vi "Execute Or Recurse.vi"(7 "Actor in":refnum<class "Actor.lvclass">, 8 "Error in":errorcluster, 10 "Msg":refnum<class "Msg.lvclass">) -> (0 "Error out":errorcluster, 2 "Msg Output":refnum<class "Msg Output.lvclass">, 5 "Actor out":refnum<class "Actor.lvclass">)   [LabVIEW 2025, in "jettl.lvlib"]
uses:
  jettl.lvlib
  Msg/Msg.lvclass
  Actor/Actor.lvclass
  Msg Output/Msg Output.lvclass
  Default Implementation.vi
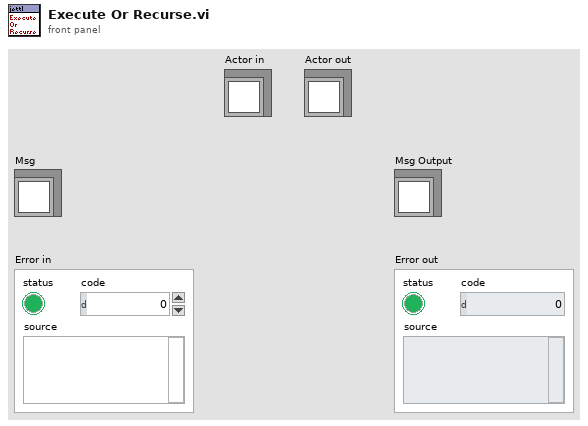
[diagram p1: front panel]
types:
  T1 = typedef "jettl.lvlib/Msgs.ctl" = set{refnum<class "Msg.lvclass">}
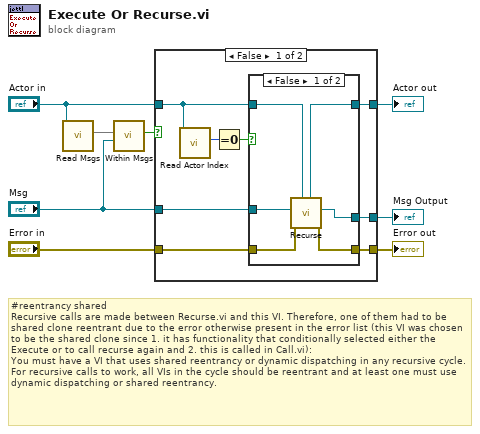
[diagram p0: block diagram]
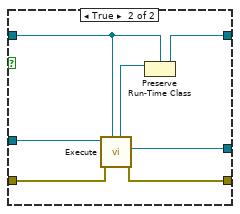
[diagram p3: hidden frame]
diagram:
  # "#reentrancy shared\nRecursive calls are made between Recurse.vi and this VI. Therefore, one of them had to be shared clone reentrant due to the error otherwise present in the error list (this VI was chosen to be the shared clone since 1. it has functionality that conditionally selected either the Execute or to call recurse again and 2. this is called in Call.vi):\nYou must have a VI that uses shared reentrancy or dynamic dispatching in any recursive cycle. For recursive calls to work, all VIs in the cycle should be reentrant and at least one must use dynamic dispatching or shared reentrancy."
  n1 = call-dynamic "Read Msgs.vi"("Actor in"="Actor in") -> ("Msgs"=w5:T1)  [unwired: 10 in]
  n2 = call "Within Msgs.vi"("Msg"="Msg", "Msgs"=w5) -> ("Within Msgs"=w8:bool)  [unwired: 9 in]
  n3 = case shown="False" w8 {
    tunnel: "Actor in" -> [w12 w29]
    tunnel: [w14 w28] -> w3
    tunnel: "Msg" -> [w16 w31]
    tunnel: [w15 w27] -> w6
    tunnel: [w13 w26] -> w2
    tunnel: "Error in" -> [w9 w25]
    frame False {
      n4 = call-dynamic "Read Actor Index.vi"("Actor in"=w12) -> ("Actor Index"=w11:i32)  [unwired: 10 in]
      n5 = Equal To 0?(x=w11) -> (x = 0?=w10:bool)
      n6 = case shown="False" w10 {
        tunnel: w16 -> [w20 _]
        tunnel: [w19 w23] -> w15
        tunnel: w12 -> [w22 w24]
        tunnel: [w21 w24] -> w14
        tunnel: [w18 _] -> w13
        tunnel: w9 -> [w17 w23]
        frame False {
          n7 = call "Recurse.vi"("Actor in"=w22, "Error in"=w17, "Msg"=w20) -> ("Error out"=w19:errorcluster, "Msg Output"=w18:refnum<class "Msg Output.lvclass">, "Actor out"=w21:refnum<class "Actor.lvclass">)  [unwired: 6 in]
        }
        frame True {
          # "Msg not implemented and this is the innermost, do nothing."
        }
      }
    }
    frame True {
      n8 = call-dynamic "Execute.vi"("Actor in"=w29, "Error in"=w25, "Msg in"=w31) -> ("Error out"=w27:errorcluster, "Msg Output"=w26:refnum<class "Msg Output.lvclass">, "Actor out"=w30:refnum<class "Actor.lvclass">)  [unwired: 6 in]
      n9 = Preserve Run-Time Class(object in=w30, 2:w29) -> (object out=w28:refnum<class "Actor.lvclass">)  [unwired: 1 in, 1 out]
    }
  }
  "Error out" <- w6
  "Actor out" <- w3
  "Msg Output" <- w2
